vi "Qualify Library Icon Core.vi"(0 "VI Reference":refnum<vi>, 11 "error in":errorcluster) -> (3 "Class?":bool, 4 "Good Library Icon":bool, 6 "Maximum Number of Rows":i32, 8 "Library Path":path, 10 "Number of Rows in Icon":i32, 14 "Icon Image":picture, 15 "error out":errorcluster)   [LabVIEW 2021, in "Text-Based VI Icon.lvlib"]
uses:
  Text-Based VI Icon.lvlib
panel:
  out "Left and Right Good (for Debugging)":bool
  out "Top and Bottom Good (for Debugging)":bool
  out "Good Frame Color (for Debugging)":bool
  out "Supported Size or Shape (for Debugging)":bool
  out "Last True Mask + 1 (for Debugging)":i32
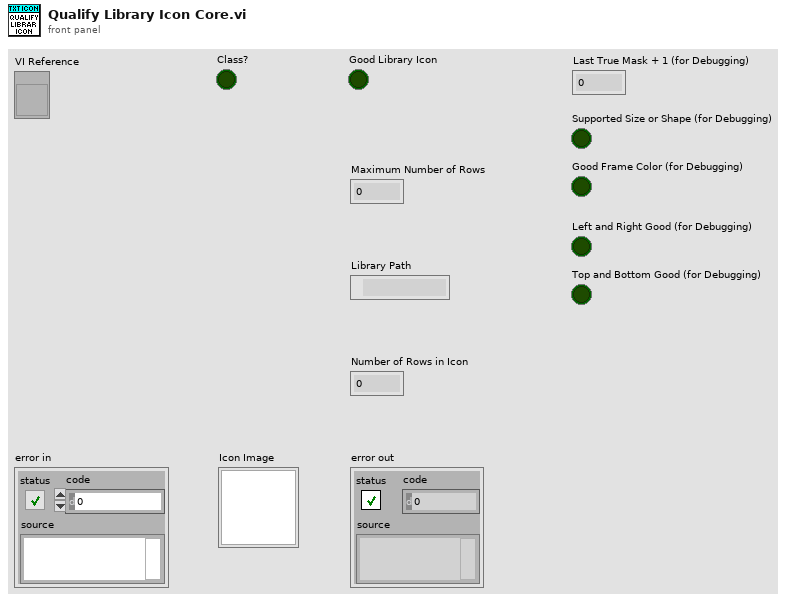
[diagram p1: front panel]
types:
  T1 = typedef "imagedata.ctl" = cluster{"image type":i32, "image depth":i32, "image":u8[], "mask":u8[], "colors":u32[], "Rectangle":cluster{"left":i16, "top":i16, "right":i16, "bottom":i16}}
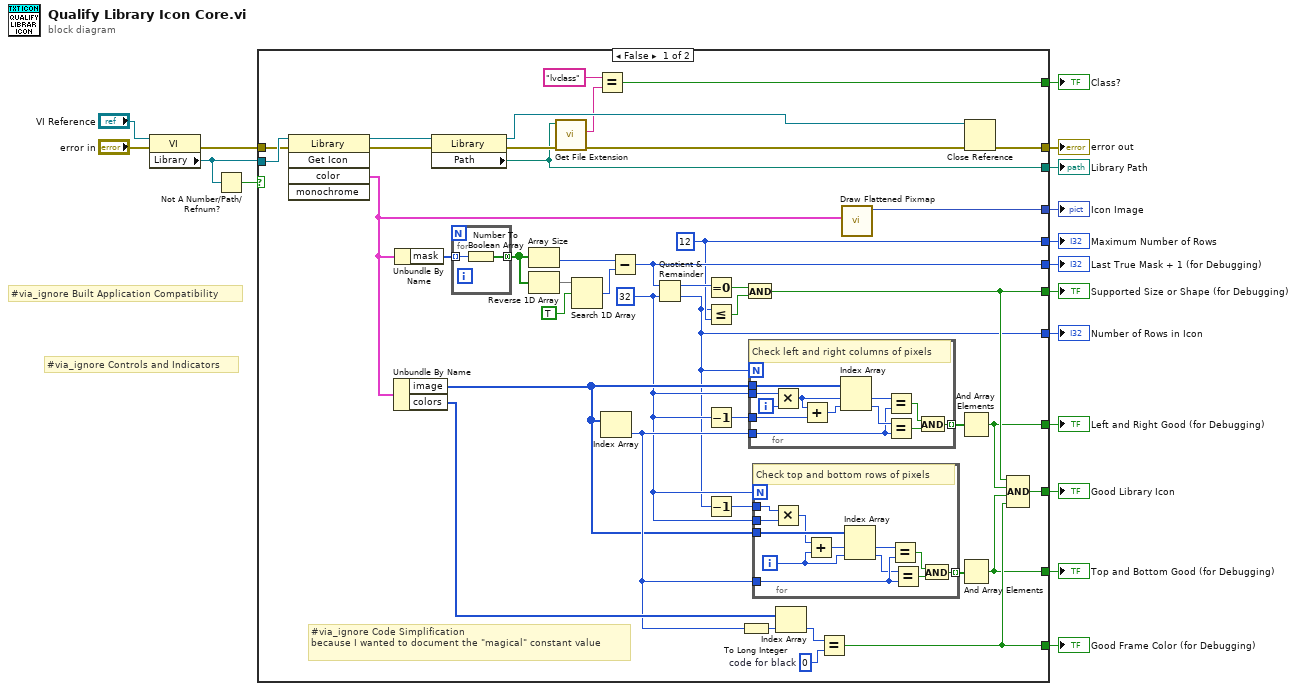
[diagram p0: block diagram]
diagram:
  # "#via_ignore Built Application Compatibility"
  # "#via_ignore Controls and Indicators"
  n1 = property class="VI"(reference="VI Reference", error in="error in") -> (error out=w15:errorcluster, "Library"=w16:refnum<vi>)  [unwired: 1 out]
  n2 = Not A Number/Path/Refnum?(number/path/refnum=w16) -> (NaN/Path/Refnum?=w17:bool)
  n3 = case shown="False" w17 {
    tunnel: w16 -> [w59 _]
    tunnel: w15 -> [w58 w86]
    tunnel: [w27 w86] -> w14
    tunnel: [w48 _] -> w13
    tunnel: [w35 _] -> w12
    tunnel: [w33 _] -> w11
    tunnel: [w32 _] -> w10
    tunnel: [w34 _] -> w9
    tunnel: [w36 _] -> w8
    tunnel: [w31 _] -> w7
    tunnel: [w20 _] -> w6
    tunnel: [w28 _] -> w3
    tunnel: [w21 _] -> w2
    tunnel: [w18 _] -> w1
    frame False {
      w46 = u32 0  # code for black
      w28 = 12 ("y")
      w37 = 32 ("y")
      # "#via_ignore Code Simplification\nbecause I wanted to document the \"magical\" constant value"
      n4 = invoke class="Library" method="Get Icon"(reference=w59, error in=w58) -> (reference out=w30:refnum<vi>, error out=w29:errorcluster, "color"=w19:T1)  [unwired: 3 in, 2 out]
      n5 = Unbundle By Name(w19) -> ("image"=w41:u8[], "colors"=w47:u32[])
      n6 = Unbundle By Name(w19) -> ("mask"=w54:u8[])
      n7 = property class="Library"(reference=w30, error in=w29) -> (reference out=w26:refnum<vi>, error out=w25:errorcluster, "Path"=w20:path)
      n8 = for {
        tunnel: w54 -> [w85] mode=indexing
        tunnel: [w84] -> w51 mode=concatenating
        n9 = Number To Boolean Array(number=w85) -> (Boolean array=w84:bool[])
      }
      n10 = Array Size(array=w51) -> (size(s)=w50:i32)
      n11 = Reverse 1D Array(array=w51) -> (reversed array=w53:bool[])
      n12 = call <vilib>:"Get File Extension.vi"("error in (no error)"=w25, "file"=w20) -> ("error out"=w24:errorcluster, "lowercase file extension"=w23:string)  [unwired: 5 in, 3 out]
      n13 = Search 1D Array(1D array=w53, element=TRUE) -> (index of element=w49:i32)  [unwired: 1 in]
      n14 = Equal?(x="lvclass", y=w23) -> (x = y?=w21:bool)
      n15 = Index Array(array=w41) -> (element=w42:u8)  [unwired: 1 in]
      n16 = Subtract(x=w50, y=w49) -> (x-y=w48:i32)
      n17 = Quotient & Remainder(x=w48, y=w37) -> (x-y*floor(x/y)=w57:i32, floor(x/y)=w18:i32)
      n18 = Equal To 0?(x=w57) -> (x = 0?=w56:bool)
      n19 = Less Or Equal?(x=w18, y=w28) -> (x <= y?=w55:bool)
      n20 = Decrement(x=w37) -> (x-1=w39:i32)
      n21 = Decrement(x=w18) -> (x-1=w43:i32)
      n22 = To Long Integer(number=w42) -> (32bit integer=w45:i32)
      n23 = And(x=w56, y=w55) -> (x .and. y?=w35:bool)
      n24 = for {
        N: w18 -> [_]
        tunnel: w42 -> [w73]
        tunnel: [w81] -> w40 mode=indexing
        tunnel: w39 -> [w79]
        tunnel: w41 -> [w77]
        tunnel: w37 -> [w75]
        i -> [w80]
        # "Check left and right columns of pixels"
        n25 = Multiply(x=w75, y=w80) -> (x*y=w72:i32)
        n26 = Add(x=w72, y=w79) -> (x+y=w74:i32)
        n27 = Index Array(array=w77, index #1=w72, index #2=w74) -> (element #1=w76:u8, element #2=w78:u8)
        n28 = Equal?(x=w76, y=w73) -> (x = y?=w83:bool)
        n29 = Equal?(x=w78, y=w73) -> (x = y?=w82:bool)
        n30 = And(x=w83, y=w82) -> (x .and. y?=w81:bool)
      }
      n31 = for {
        N: w37 -> [_]
        tunnel: w41 -> [w71]
        tunnel: w43 -> [w70]
        tunnel: w42 -> [w65]
        tunnel: [w61] -> w44 mode=indexing
        tunnel: w37 -> [w60]
        i -> [w67]
        # "Check top and bottom rows of pixels"
        n32 = Multiply(x=w70, y=w60) -> (x*y=w69:i32)
        n33 = Add(x=w69, y=w67) -> (x+y=w68:i32)
        n34 = Index Array(array=w71, index #1=w68, index #2=w67) -> (element #1=w66:u8, element #2=w64:u8)
        n35 = Equal?(x=w66, y=w65) -> (x = y?=w63:bool)
        n36 = Equal?(x=w64, y=w65) -> (x = y?=w62:bool)
        n37 = And(x=w63, y=w62) -> (x .and. y?=w61:bool)
      }
      n38 = Index Array(array=w47, index=w45) -> (element=w38:u32)
      n39 = Equal?(x=w38, y=w46) -> (x = y?=w33:bool)
      n40 = call <vilib>:"Draw Flattened Pixmap.vi"("image data"=w19) -> ("new picture"=w36:picture)  [unwired: 8 in]
      n41 = And Array Elements(Boolean array=w40) -> (logical AND=w34:bool)
      n42 = And Array Elements(Boolean array=w44) -> (logical AND=w32:bool)
      n43 = Close Reference(reference=w26, error in (no error)=w24) -> (error out=w27:errorcluster)
      n44 = Compound Arithmetic op=AND(w35, w34, w32, w33) -> (w31:bool)
    }
    frame True {
    }
  }
  "error out" <- w14
  "Last True Mask + 1 (for Debugging)" <- w13
  "Supported Size or Shape (for Debugging)" <- w12
  "Good Frame Color (for Debugging)" <- w11
  "Top and Bottom Good (for Debugging)" <- w10
  "Left and Right Good (for Debugging)" <- w9
  "Icon Image" <- w8
  "Good Library Icon" <- w7
  "Library Path" <- w6
  "Maximum Number of Rows" <- w3
  "Class?" <- w2
  "Number of Rows in Icon" <- w1
